vi "constants.vi"() -> ()   [LabVIEW 2018]
panel:
  out "Legal_Drivers":string[](array[string])
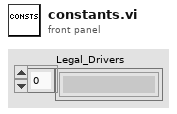
[diagram p1: front panel]
diagram:
